vi "Test plot array data.vi"() -> ()   [LabVIEW 2015]
panel:
  out "Position Plot":i32[](graph)
  out "Data Array plot":u8[](graph)
  in  "Full Data Array":u8[][](array[numeric])=array300x1009[302700 elements]
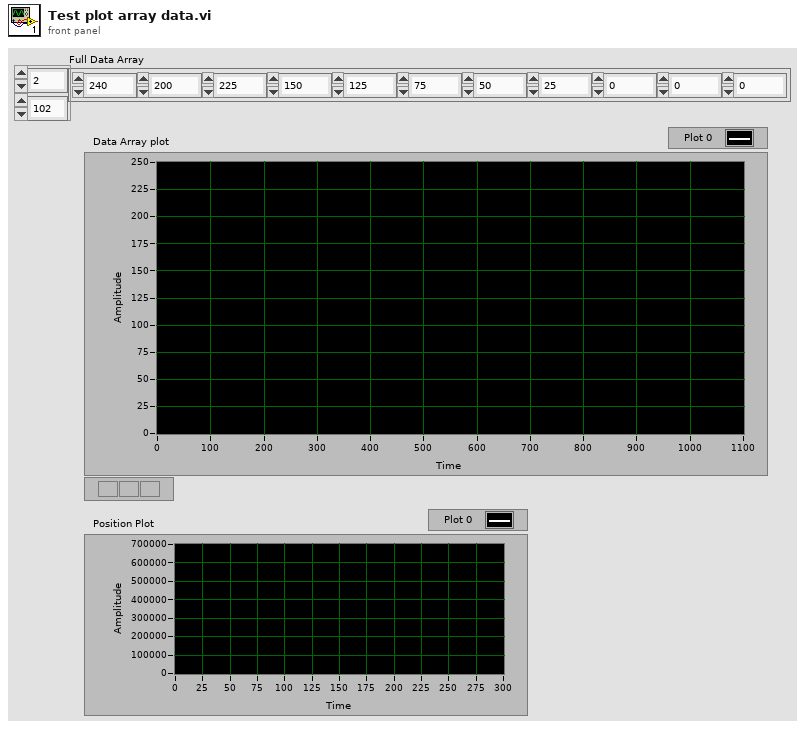
[diagram p1: front panel]
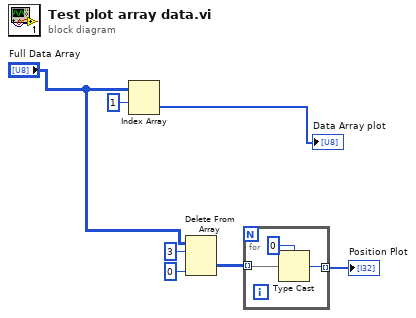
[diagram p0: block diagram]
diagram:
  n1 = Index Array(array="Full Data Array", index (row)=1) -> (element=→"Data Array plot":u8[])  [unwired: 1 in]
  n2 = Delete From Array(array="Full Data Array", length=3, index (col)=0 ("disabled index (col)")) -> (deleted portion=w3:u8[][])  [unwired: 1 in, 1 out]
  n3 = for {
    tunnel: w3 -> [w10] mode=indexing
    tunnel: [w8] -> w1 mode=indexing
    n4 = Type Cast(type=0, x=w10) -> (*(type *) &x=w8:i32)
  }
  "Position Plot" <- w1
